vi "Read Publish Data.vi"(8 "error in (no error)":errorcluster, 10 "Write Data?":bool=TRUE, 11 "Model in":refnum<class "Model.lvclass">) -> (0 "error out":errorcluster, 3 "Model out":refnum<class "Model.lvclass">)   [LabVIEW 2016, in "Model.lvclass"]
uses:
  Model.lvclass
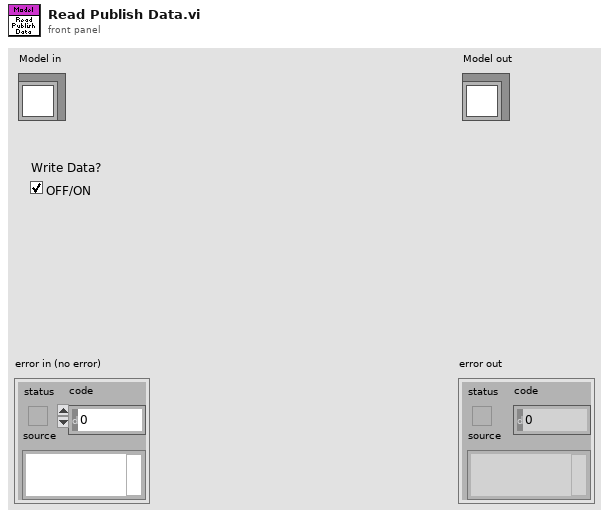
[diagram p1: front panel]
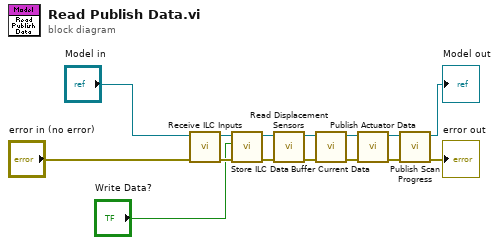
[diagram p0: block diagram]
diagram:
  n1 = call "Receive ILC Inputs.vi"("error in (no error)"="error in (no error)", "Model in"="Model in") -> ("error out"=w7:errorcluster, "Model out"=w14:refnum<class "Model.lvclass">)  [unwired: 8 in]
  n2 = call "Store ILC Data.vi"("error in (no error)"=w7, "Write Data?"="Write Data?", "Model in"=w14) -> ("error out"=w6:errorcluster, "Model out"=w13:refnum<class "Model.lvclass">)  [unwired: 7 in]
  n3 = call "Read Displacement Sensors.vi"("error in (no error)"=w6, "Model in"=w13) -> ("error out"=w5:errorcluster, "Model out"=w12:refnum<class "Model.lvclass">)  [unwired: 8 in]
  n4 = call "Buffer Current Data.vi"("error in (no error)"=w5, "Model in"=w12) -> ("error out"=w4:errorcluster, "Model out"=w11:refnum<class "Model.lvclass">)  [unwired: 8 in]
  n5 = call "Publish Actuator Data.vi"("error in (no error)"=w4, "Model in"=w11) -> ("error out"=w3:errorcluster, "Model out"=w10:refnum<class "Model.lvclass">)  [unwired: 8 in]
  n6 = call "Publish Scan Progress.vi"("error in (no error)"=w3, "Model in"=w10) -> ("error out"=→"error out":errorcluster, "Model out"=→"Model out":refnum<class "Model.lvclass">)  [unwired: 8 in]
